vi "Get Measurement Type.vi"(8 "error in (no error)":errorcluster, 11 "DCLeakage in":refnum<class "DCLeakage.lvclass">=refnum) -> (0 "error out":errorcluster, 2 "Measurement Type":string="DCPower", 3 "DCLeakage out":refnum<class "DCLeakage.lvclass">)   [LabVIEW 2018, in "DCLeakage.lvlib" / "DCLeakage.lvclass"]
uses:
  DCLeakage.lvclass
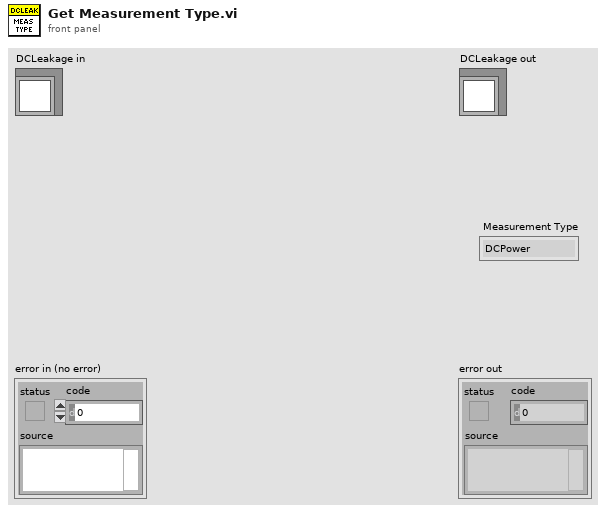
[diagram p1: front panel]
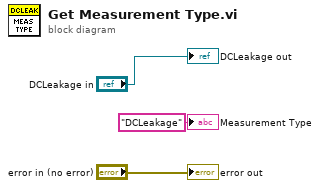
[diagram p0: block diagram]
diagram:
  "error out" <- "error in (no error)"
  "DCLeakage out" <- "DCLeakage in"
  "Measurement Type" <- "DCLeakage" ("Measurement Type")
